vi "Init Position_LVDT_AI Channel.vi"(8 "error in":errorcluster, 9 "Position_LVDT_Properties":T1={"Minimum Value"=-0.1, "Maximum Value"=0.1, "Excitation Source"=10200, "Excitation Wire Mode"=4, "Excitation Frequency"=2500.0, "Excitation Value"=1.0, "Units"=10219, "Sensitivity"=50.0, "Sensitivity Units"=12506, "Excitation Sense"=16095} {"Excitation Sense" items=["Local"=16095, "Remote"=16096]; "Excitation Source" items=["Internal"=10200, "External"=10167, "None"=10230]; "Excitation Wire Mode" items=["4-Wire"=4, "5-Wire"=5, "6-Wire"=6]; "Units" items=["Meters"=10219, "Inches"=10379, "From Custom Scale"=10065]; "Sensitivity Units" items=["mVolts/Volt/mMeter"=12506, "mVolts/Volt/0.001 Inch"=12505]}, 10 "physical channel":tag, 11 "task in":refnum<k21>) -> (0 "error out":errorcluster, 3 "task out":refnum<k21>)   [LabVIEW 2020, in "NI PXIe-4340 Engine.lvlib"]
uses:
  NI PXIe-4340 Engine.lvlib
  Shared/Position_LVDT_Properties.ctl
  <vilib>/DAQmx/create/channels.llb/DAQmx Create Channel (AI-Position-LVDT).vi
  <resource>/objmgr/daqmx.rc
  Shared/NI PXIe-4340 Shared.lvlib
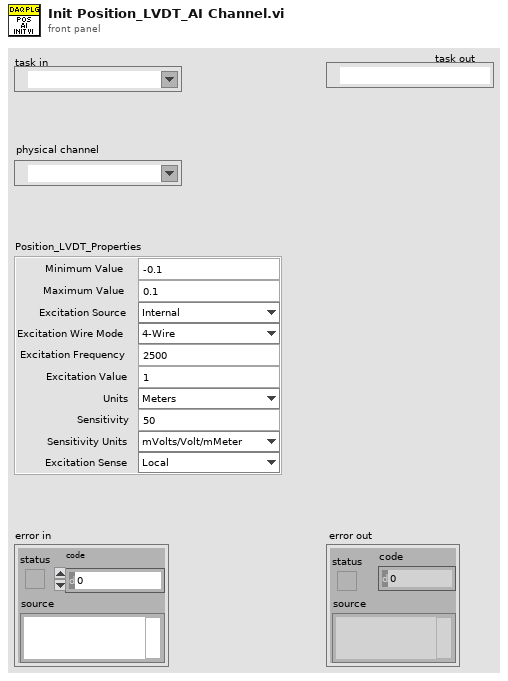
[diagram p1: front panel]
types:
  T1 = typedef "NI PXIe-4340 Shared.lvlib/Position_LVDT_Properties.ctl" = cluster{"Minimum Value":dbl, "Maximum Value":dbl, "Excitation Source":i32, "Excitation Wire Mode":i32, "Excitation Frequency":dbl, "Excitation Value":dbl, "Units":i32, "Sensitivity":dbl, "Sensitivity Units":i32, "Excitation Sense":i32}
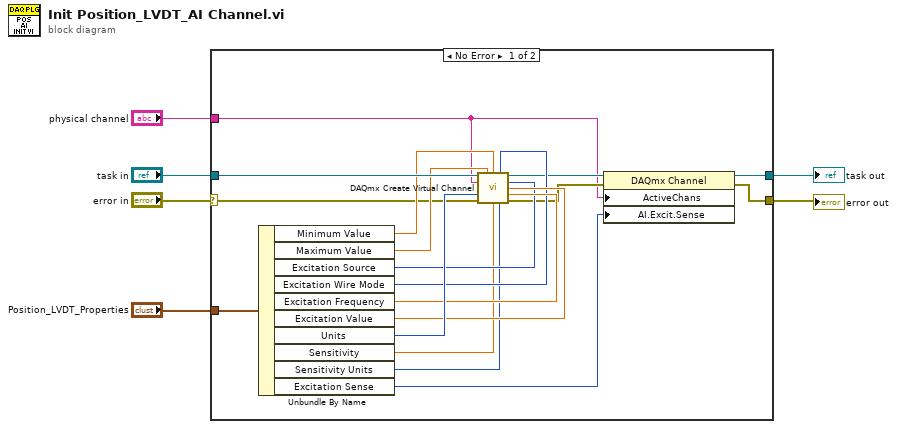
[diagram p0: block diagram]
diagram:
  n1 = case shown="No Error" "error in" {
    selector: "error in" -> [w8 w26]
    tunnel: [w14 w25] -> w6
    tunnel: [w12 w26] -> w2
    tunnel: "task in" -> [w24 w25]
    tunnel: "physical channel" -> [w7 _]
    tunnel: "Position_LVDT_Properties" -> [w9 _]
    frame No Error {
      n2 = Unbundle By Name(w9) -> ("Minimum Value"=w22:dbl, "Maximum Value"=w23:dbl, "Excitation Source"=w18:i32, "Excitation Wire Mode"=w17:i32, "Excitation Frequency"=w19:dbl, "Excitation Value"=w20:dbl, "Units"=w21:i32, "Sensitivity"=w16:dbl, "Sensitivity Units"=w15:i32, "Excitation Sense"=w10:i32)
      n3 = call-poly <vilib>:"DAQmx Create Virtual Channel.vi"("task in"=w24, "maximum value"=w23, "minimum value"=w22, "voltage excitation wire mode"=w17, "physical channels"=w7, "voltage excitation source"=w18, "voltage excitation value"=w20, "units"=w21, "voltage excitation frequency"=w19, "error in"=w8, "sensitivity"=w16, "sensitivity units"=w15) -> ("task out"=w11:refnum<k21>, "error out"=w13:errorcluster)  [unwired: 2 in]
      n4 = property class="DAQmx Channel"(reference=w11, error in=w13, "ActiveChans"=w7, "AI.Excit.Sense"=w10) -> (reference out=w14:refnum<k21>, error out=w12:errorcluster)
    }
    frame Error {
    }
  }
  "task out" <- w6
  "error out" <- w2
